vi "Define Columns.vi"(10 "Enum Array":refnum<vi>[](array[refnum])) -> (2 "Column Definition":T1[](array[typedef]) {"MinWidth" min=2 step=1; "AutoSizeMode" items=["None"=1, "ColumnHeader"=2, "AllCellsExceptHeader"=4, "AllCells"=6, "DisplayedCellsExceptHeader"=8, "DisplayedCells"=10, "Fill"=16]; "FillWeight" min=1 max=100})   [LabVIEW 2013, in "Scan Engine editor node.lvclass"]
doc: "This VI defines the columns that will be used in the table. You can specify the column type and the dimensions if the columns."
uses:
  Scan Engine editor node.lvclass
  <vilib>/NI/DCAF/Tag Editor Core/Table API/Column/Column Descriptor.ctl
  <vilib>/NI/DCAF/Tag Editor Core/Table API/Column/Column.lvclass
  <vilib>/NI/DCAF/Tag Editor Core/Table API/Column/Column Type.ctl
  <vilib>/NI/Tag Bus/tag/Data Type.ctl
  <vilib>/NI/DCAF/Tag Editor Core/Table API/Table Manager/Call Back Ref Type Def.ctl
  <vilib>/NI/DCAF/Tag Editor Core/Configuration Editor/Classes/Engine Parent/Engine Parent Editor Node.lvclass
  <vilib>/NI/DCAF/Tag Editor Core/Configuration Editor/Classes/Module editor node/module editor node.lvclass
  <vilib>/NI/Tag Bus/tag/tag descriptor.lvclass
  <vilib>/NI/DCAF/Tag Editor Core/Table API/Mapping Column/Mapping Column.lvclass
  <vilib>/NI/DCAF/Tag Editor Core/Table API/String Column/String Column.lvclass
  <vilib>/NI/DCAF/Tag Editor Core/Table API/Listbox Enum Column/List Box Enum Column.lvclass
  <vilib>/NI/DCAF/Tag Editor Core/Table API/Table Manager/Table Manager.lvclass
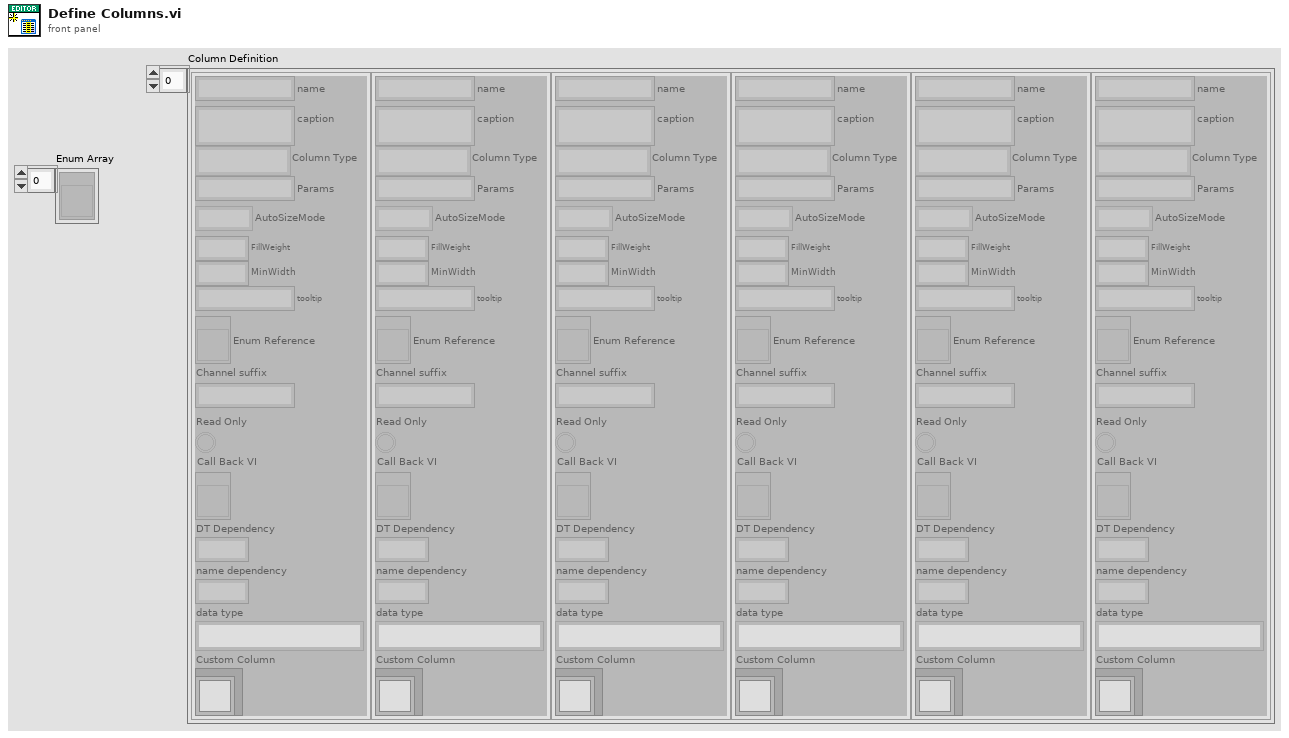
[diagram p1: front panel]
types:
  T1 = typedef "Table Manager.lvlib/Column.lvclass/Column Descriptor.ctl" = cluster{"name":string, "caption":string, "Column Type":T2, "Params":string, "AutoSizeMode":i32, "FillWeight":sgl, "MinWidth":u32, "tooltip":string, "Enum Reference":refnum<vi>, "Channel suffix":string, "Read Only":bool, "Call Back VI":T3, "DT Dependency":i32, "name dependency":i32, "data type":T4, "Custom Column":refnum<class "Column.lvclass">}
  T2 = typedef "Table Manager.lvlib/Column.lvclass/Column Type.ctl" = enum16{"String", "Mapping", "Enum", "Custom"}
  T3 = typedef "Table Manager.lvlib/Table Manager.lvclass/Call Back Ref Type Def.ctl" = refnum<vi>
  T4 = typedef "tag bus.lvlib/tag descriptor.lvclass/Data Type.ctl" = enum16{"Double", "Single", "I64", "I32", "I16", "I8", "U64", "U32", "U16", "U8", "Boolean", "String", "Array of Double", "Array of Single", "Array of I64", "Array of I32", "Array of I16", "Array of I8", "Array of U64", "Array of U32", "Array of U16", "Array of U8", "Array of Boolean", "Array of String"}
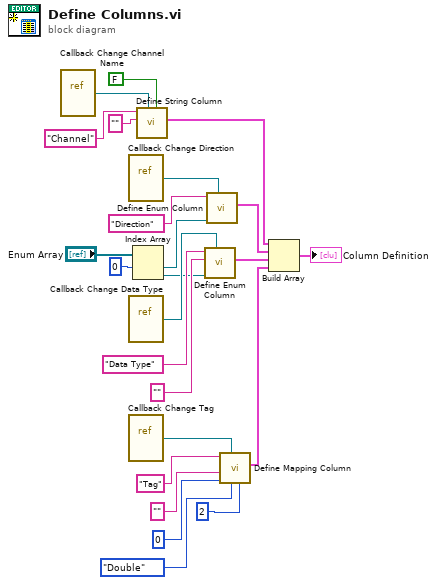
[diagram p0: block diagram]
diagram:
  n1 = vi-ref "Callback Change Channel Name.vi"() -> (w11:refnum<vi>)
  n2 = vi-ref "Callback Change Direction.vi"() -> (w7:refnum<vi>)
  n3 = vi-ref "Callback Change Data Type.vi"() -> (w4:refnum<vi>)
  n4 = vi-ref "Callback Change Tag.vi"() -> (w23:refnum<vi>)
  n5 = Index Array(array="Enum Array", index #1=0 ("index")) -> (element #1=w8:refnum<vi>, element #2=w1:refnum<vi>)  [unwired: 1 in]
  n6 = call <vilib>:"Define String Column.vi"("Read Only (F)"=FALSE ("Read Only"), "Call Back VI"=w11, "Caption"="", "Name"="Channel" ("name")) -> ("Column Descriptor out"=w13:T1)  [unwired: 7 in]
  n7 = call <vilib>:"Define Enum Column.vi"("Call Back VI"=w4, "Enum Reference"=w1, "Caption"="", "Name"="Data Type" ("name")) -> ("Column Descriptor out"=w2:T1)  [unwired: 7 in]
  n8 = call <vilib>:"Define Enum Column.vi"("Call Back VI"=w7, "Enum Reference"=w8, "Name"="Direction" ("name")) -> ("Column Descriptor out"=w6:T1)  [unwired: 8 in]
  n9 = call <vilib>:"Define Mapping Column.vi"("DT Dependency (-1)"=2 ("DT Dependency"), "data type"=Data_Type."Double", "Call Back VI"=w23, "name dependency"=0, "Channel suffix"="" ("string"), "name"="Tag") -> ("Column Descriptor out"=w10:T1)  [unwired: 5 in]
  n10 = Build Array(w13, w6, w2, w10) -> (→"Column Definition":T1[])
